vi "Histogram Equalization.vi"() -> ()   [LabVIEW 2014]
doc: "Use this template to build a VI to use as a subVI."
uses:
  <vilib>/vision/NI_Vision_Development_Module.lvlib
panel:
  out "H-Cuml-Dst":T1(graph)
  out "H-Dst":T1(graph)
  out "H-Cuml-Src":T1(graph)
  out "Dst":T2(plugin-control)
  out "H-Src":T1(graph)
  out "Src":T2(plugin-control)
  # ":: MVi Framework V1.0 ::\nAuthor:Gaoke Yang\nEmail: gaoke.yang@yahoo.com\nWeb: www.mvicontrol.com\nCopyright (C) 2015, MVI Technologies All Rights Reserved"
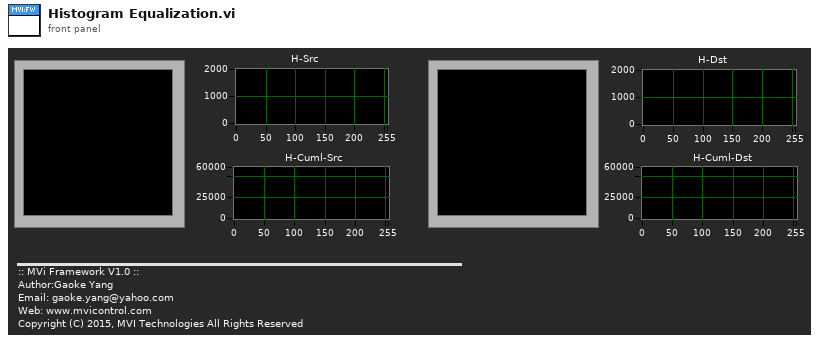
[diagram p1: front panel]
types:
  T1 = cluster{"Starting Value":sgl, "Incremental Value":sgl, "Histogram":u32[]}
  T2 = typedef "IMAQ Image.ctl" = refnum<image>
  T3 = typedef "Image Type" = u32
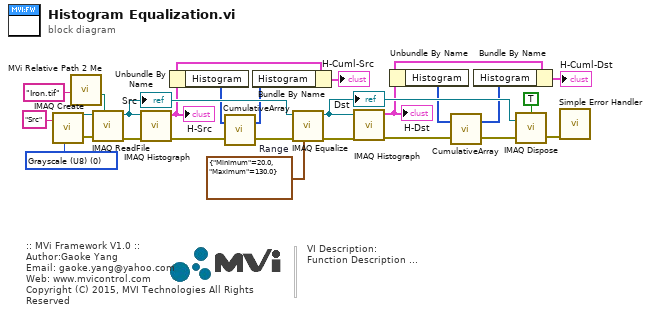
[diagram p0: block diagram]
diagram:
  w14 = cluster{"Minimum":sgl, "Maximum":sgl} {"Minimum"=20.0, "Maximum"=130.0}  # Range
  w15 = T3 0 items=["Grayscale (U8)", "Grayscale (I16)", "Grayscale (SGL)", "Complex (CSG)", "RGB (U32)", "HSL (U32)", "RGB (U64)", "Grayscale (U16)"] ("Image Type")
  # "VI Description:\nFunction Description ..."
  # ":: MVi Framework V1.0 ::\nAuthor:Gaoke Yang\nEmail: gaoke.yang@yahoo.com\nWeb: www.mvicontrol.com\nCopyright (C) 2015, MVI Technologies All Rights Reserved"
  n1 = call "IMAQ Create"("Image Name"="Src" ("name or relative path"), "Image Type"=w15) -> ("New Image"=w20:T2, "error out"=w19:errorcluster)  [unwired: 2 in, 1 out]
  n2 = call "MVi Relative Path 2 Me.vi"("Relative Path"="Iron.tif" ("name or relative path")) -> ("Appended Dir"=w21:path)  [unwired: 5 in, 1 out]
  n3 = call "IMAQ ReadFile"("File Path"=w21, "error in (no error)"=w19, "Image"=w20) -> ("error out"=w18:errorcluster, "Image Out"=w13:T2)  [unwired: 4 in, 3 out]
  "Src" <- w13
  n4 = call "IMAQ Histograph"("error in (no error)"=w18, "Image"=w13) -> ("error out"=w8:errorcluster, "Histogram Graph"=w5:T1)  [unwired: 6 in, 2 out]
  "H-Src" <- w5
  n5 = Unbundle By Name(w5) -> ("Histogram"=w7:u32[])
  n6 = call "CumulativeArray.vi"("error in"=w8, "ArrayIn"=w7) -> ("error out"=w3:errorcluster, "ArrayOut"=w6:u32[])
  n7 = Bundle By Name(cluster=w5, "Histogram"=w6) -> (→"H-Cuml-Src":T1)
  n8 = call "IMAQ Equalize"("Range"=w14, "error in (no error)"=w3, "Image Src"=w13) -> ("error out"=w17:errorcluster, "Image Dst Out"=w16:T2)  [unwired: 7 in]
  "Dst" <- w16
  n9 = call "IMAQ Histograph"("error in (no error)"=w17, "Image"=w16) -> ("error out"=w10:errorcluster, "Histogram Graph"=w2:T1)  [unwired: 6 in, 2 out]
  "H-Dst" <- w2
  n10 = Unbundle By Name(w2) -> ("Histogram"=w12:u32[])
  n11 = call "CumulativeArray.vi"("error in"=w10, "ArrayIn"=w12) -> ("error out"=w9:errorcluster, "ArrayOut"=w11:u32[])
  n12 = Bundle By Name(cluster=w2, "Histogram"=w11) -> (→"H-Cuml-Dst":T1)
  n13 = call "IMAQ Dispose"("All Images? (No)"=TRUE, "Image"=w16, "error in (no error)"=w9) -> ("error out"=w22:errorcluster)  [unwired: 3 out]
  n14 = call <vilib>:"Simple Error Handler.vi"("error in (no error)"=w22) -> ()  [unwired: 1 in, 8 out]
